vi "FuturePose.vi"(10 "IA State Input":T1) -> (2 "output cluster":T1={"our_robots"=[], "enemy_robots"=[], "balls"=[], "geometry"={"line_width"=0, "field_length"=0, "field_width"=0, "boundary_width"=0, "referee_width"=0, "goal_width"=0, "goal_depth"=0, "goal_wall_width"=0, "center_circle_radius"=0, "defense_radius"=0, "defense_stretch"=0, "free_kick_from_defense_dist"=0, "penalty_spot_from_field_line_dist"=0, "penalty_line_from_spot_dist"=0}, "IA Judge"={"stage"="", "command"="", "our_goalie_id"=0.0, "enemy_goalie_id"=0.0, "command enum"=enum."Halt", "Time"=enum."Azul"}, "Received Timestamp"=timestamp(0 s since 1904-01-01), "Events"={"Touch"=FALSE, "Ball out"=FALSE, "id touch"=0.0, "Ball out of \nVision"=FALSE, "Ball inside \nGoalie area"=FALSE, "Robot not responding"=FALSE, "Robots responding status"=[1.0, 1.0, 1.0, 1.0, 1.0, 1.0], "Enemy Ball \nPossession"=FALSE, "Pass State"=FALSE, "id end of pass"=0.0, "Kick"=FALSE, "Id ini Possession"=0.0, "Ball Possesion"=FALSE, "Id Possesion"=0.0, "Direct Kick"=FALSE, "2nd Strk Ativo"=FALSE}})   [LabVIEW 2020]
uses:
  SSL Detection Frame Simple Estimator Cameras VelCmd Folder/Core/AI Input.ctl
  Controls/AI Robot.ctl
  Controls/Functions Enum.ctl
  Controls/AttackerStates.ctl
  Controls/PathDests.ctl
  Controls/PathDest.ctl
  SSL Detection Frame Simple Estimator Cameras VelCmd Folder/Core/AI Ball.ctl
  SSL Detection Frame Simple Estimator Cameras VelCmd Folder/Core/Field Size.ctl
  SSL Detection Frame Simple Estimator Cameras VelCmd Folder/Core/AI Judge.ctl
  Communication_class/Paths/MessageAI_State Folder/Intel/Command Enum.ctl
  SSL Detection Frame Simple Estimator Cameras VelCmd Folder/Util/Events/Events.ctl
  <vilib>/Analysis/coordinate.llb/2D Cartesian Coordinate Rotation (Scalar).vi
  <vilib>/Analysis/NI_AALPro.lvlib
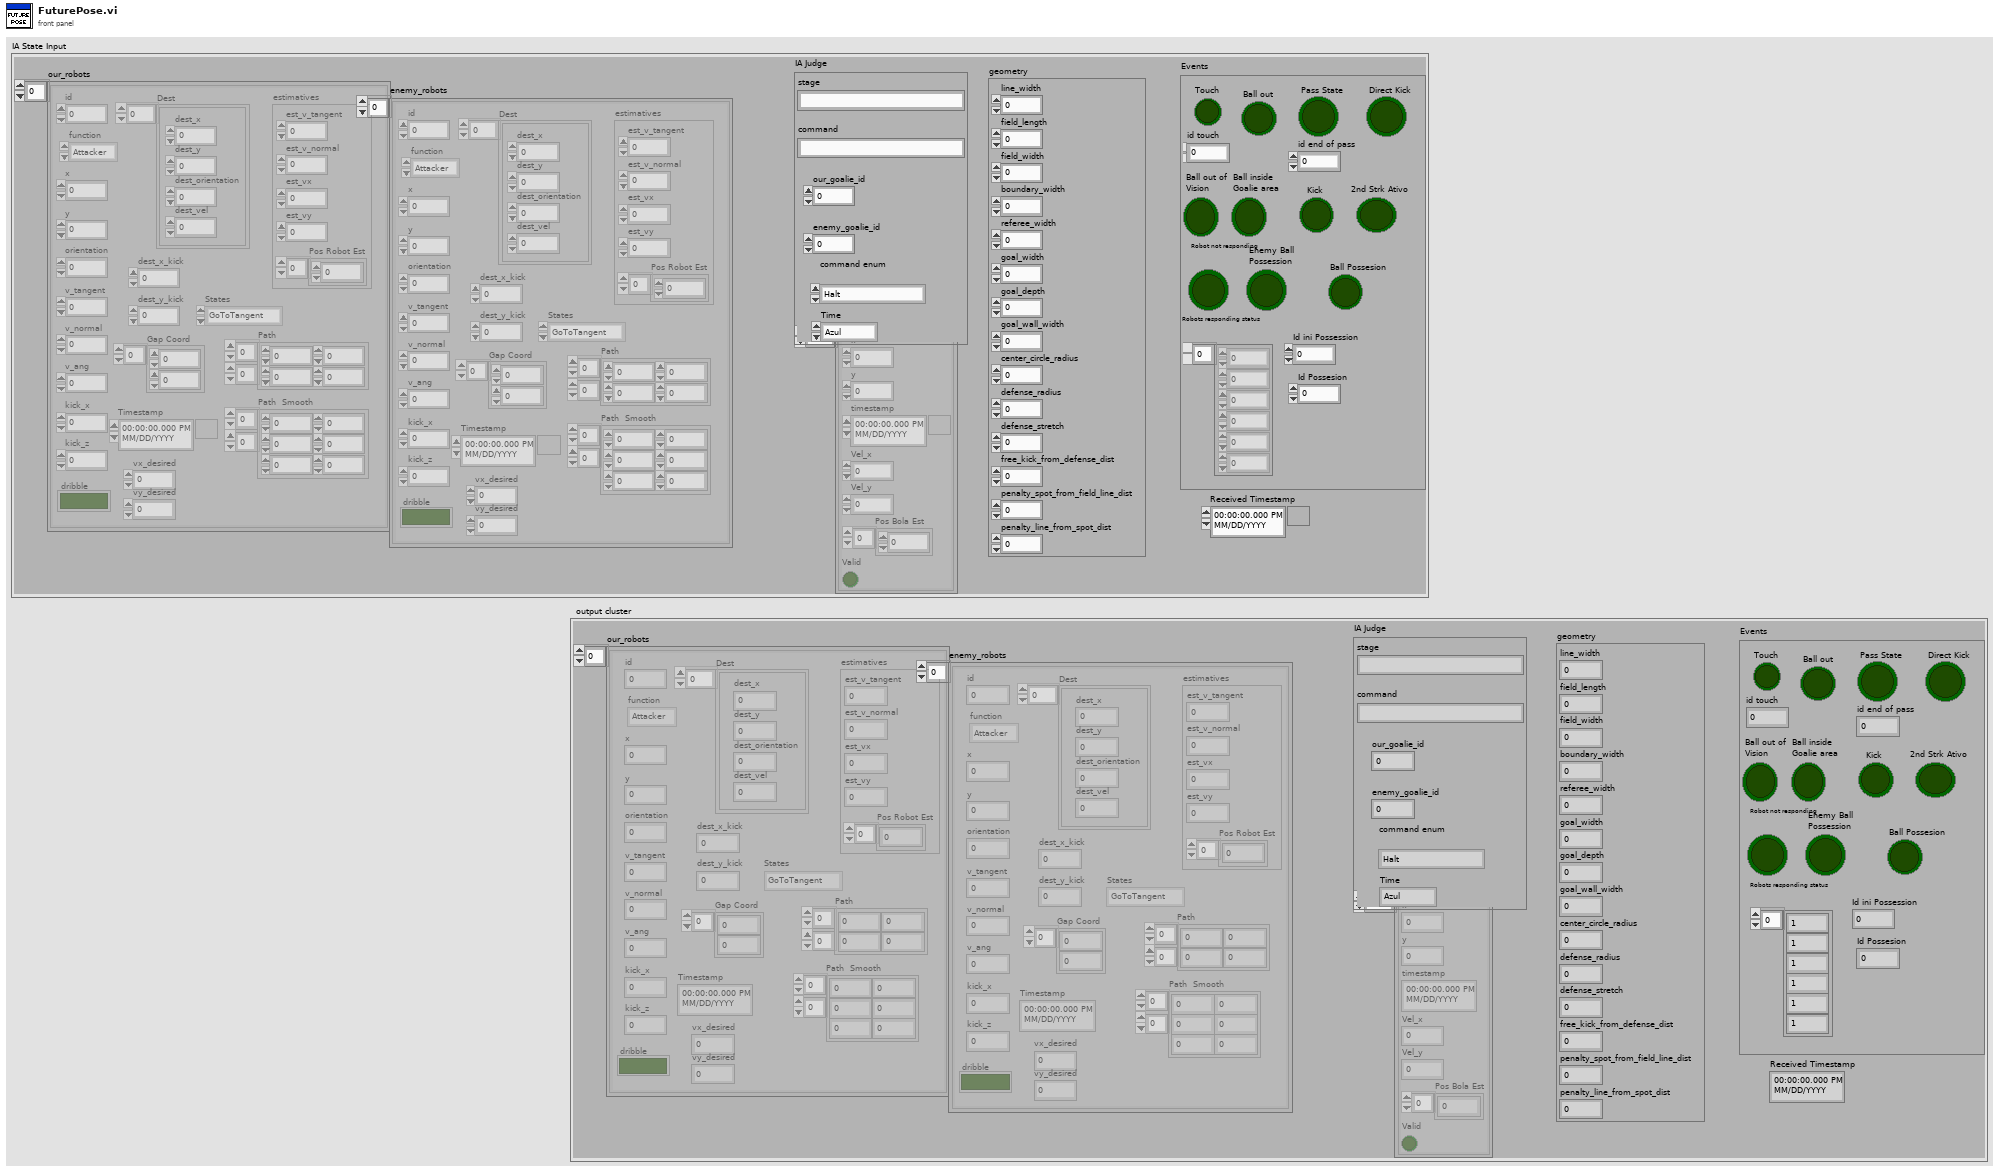
[diagram p1: front panel]
types:
  T1 = typedef "AI Input.ctl" = cluster{"our_robots":T2[], "enemy_robots":T2[], "balls":T7[], "geometry":T8, "IA Judge":T9, "Received Timestamp":timestamp, "Events":T11}
  T2 = typedef "AI Robot.ctl" = cluster{"id":u32, "function":T3, "x":dbl, "y":dbl, "orientation":dbl, "v_tangent":dbl, "v_normal":dbl, "v_ang":dbl, "kick_x":dbl, "kick_z":dbl, "dribble":bool, "Timestamp":timestamp, "estimatives":cluster{"est_v_tangent":dbl, "est_v_normal":dbl, "est_vx":dbl, "est_vy":dbl, "Pos Robot Est":dbl[]}, "dest_x_kick":dbl, "dest_y_kick":dbl, "Gap Coord":dbl[], "States":T4, "Path ":dbl[][], "Path  Smooth":dbl[][], "Dest":T5, "vx_desired":dbl, "vy_desired":dbl}
  T3 = typedef "Functions Enum.ctl" = enum16{"2nd Striker", "Attacker", "Goalie", "Defender", "Striker", "Goto 0", "Dummy", "Kicker", "ZigZag 0", "ZigZag 1", "ZigZag 2", "ZigZag 3", "ZigZag 4", "ZigZag 5", "ZigZag 6", "ZigZag 7", "ZigZag 8", ""}
  T4 = typedef "AttackerStates.ctl" = enum16{"Pass", "GoToTangent", "BallGetting", "GoToKick", ""}
  T5 = typedef "PathDests.ctl" = T6[]
  T6 = typedef "PathDest.ctl" = cluster{"dest_x":dbl, "dest_y":dbl, "dest_orientation":dbl, "dest_vel":dbl}
  T7 = typedef "AI Ball.ctl" = cluster{"x":dbl, "y":dbl, "timestamp":timestamp, "Vel_x":dbl, "Vel_y":dbl, "Pos Bola Est":dbl[], "Valid":bool}
  T8 = typedef "Field Size.ctl" = cluster{"line_width":u32, "field_length":u32, "field_width":u32, "boundary_width":u32, "referee_width":u32, "goal_width":u32, "goal_depth":u32, "goal_wall_width":u32, "center_circle_radius":u32, "defense_radius":u32, "defense_stretch":u32, "free_kick_from_defense_dist":u32, "penalty_spot_from_field_line_dist":u32, "penalty_line_from_spot_dist":u32}
  T9 = typedef "AI Judge.ctl" = cluster{"stage":string, "command":string, "our_goalie_id":dbl, "enemy_goalie_id":dbl, "command enum":T10, "Time":enum16{"Azul", "Amarelo"}}
  T10 = typedef "Command Enum.ctl" = enum16{"Halt", "Stop", "Force Start", "PKA Normal Start", "Prepare Kickoff Ally", "PKE Normal Start", "Prepare Kickoff Enemy", "Prepare Penalty Ally", "PPA Normal Start", "Prepare Penalty Enemy", "PPE Normal Start", "Direct Free Enemy", "Direct Free Ally", "Indirect Free Enemy", "Indirect Free Ally", "Timeout Enemy", "Timeout Ally", "Goal Enemy", "Goal Ally", "Ball Placement Enemy", "Ball Placement Ally", "Normal Half Time", "Extra Time Break", "Extra Half Time", "None", "Post Game"}
  T11 = typedef "Events.ctl" = cluster{"Touch":bool, "Ball out":bool, "id touch":dbl, "Ball out of \nVision":bool, "Ball inside \nGoalie area":bool, "Robot not responding":bool, "Robots responding status":dbl[], "Enemy Ball \nPossession":bool, "Pass State":bool, "id end of pass":dbl, "Kick":bool, "Id ini Possession":dbl, "Ball Possesion":bool, "Id Possesion":dbl, "Direct Kick":bool, "2nd Strk Ativo":bool}
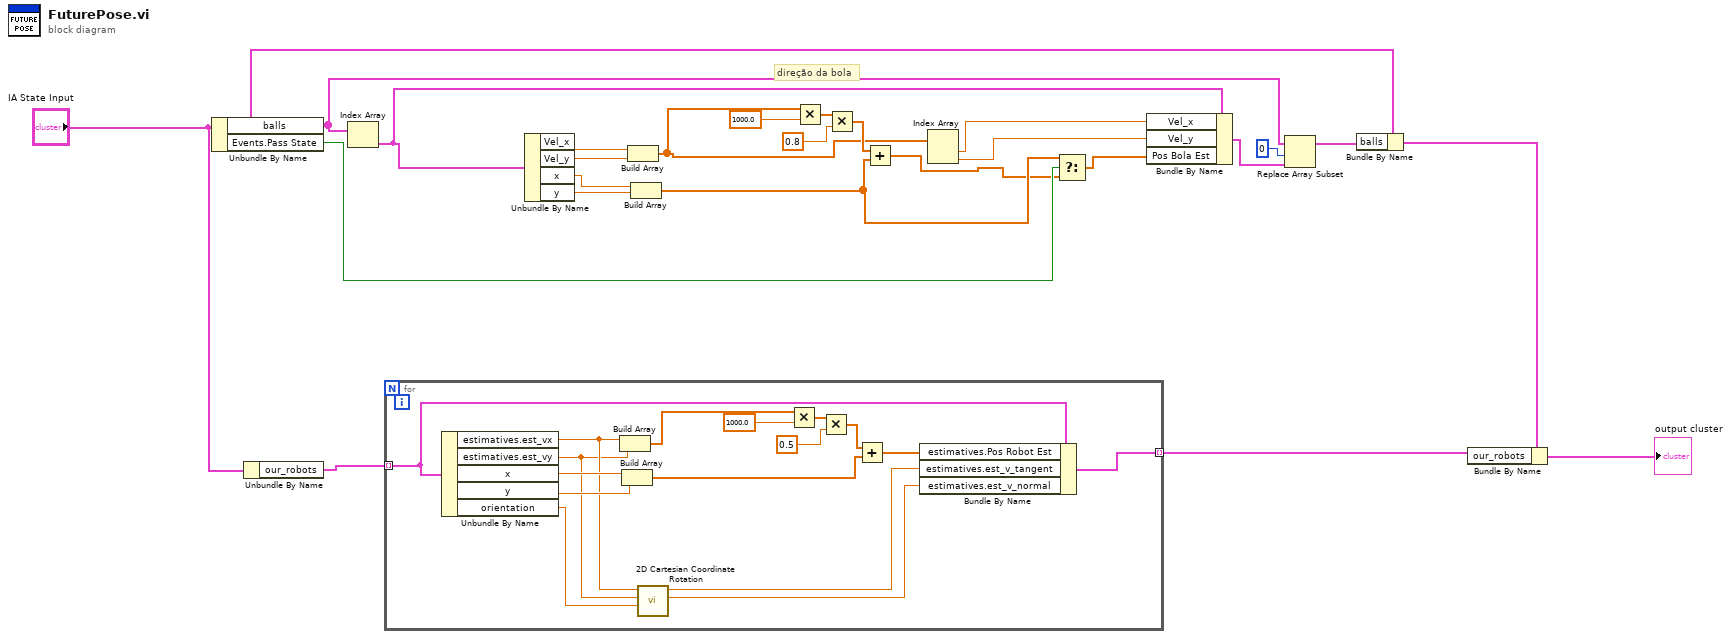
[diagram p0: block diagram]
diagram:
  # "direção da bola"
  n1 = Unbundle By Name("IA State Input") -> ("balls"=w21:T7[], "Events.Pass State"=w7:bool)
  n2 = Unbundle By Name("IA State Input") -> ("our_robots"=w6:T2[])
  n3 = Index Array(array=w21) -> (element=w23:T7)  [unwired: 1 in]
  n4 = for {
    tunnel: w6 -> [w33] mode=indexing
    tunnel: [w31] -> w5 mode=indexing
    n5 = Unbundle By Name(w33) -> ("estimatives.est_vx"=w30:dbl, "estimatives.est_vy"=w29:dbl, "x"=w35:dbl, "y"=w34:dbl, "orientation"=w28:dbl)
    n6 = Build Array(w30, w29) -> (w37:dbl[])
    n7 = Build Array(w35, w34) -> (w36:dbl[])
    n8 = call-poly <vilib>:"2D Cartesian Coordinate Rotation.vi"("theta"=w28, "y"=w29, "x"=w30) -> ("y out"=w26:dbl, "x out"=w27:dbl)  [unwired: 6 in, 1 out]
    n9 = Multiply(x=w37, y=1000.0) -> (x*y=w39:dbl[])
    n10 = Multiply(x=w39, y=0.5) -> (x*y=w40:dbl[])
    n11 = Add(x=w40, y=w36) -> (x+y=w32:dbl[])
    n12 = Bundle By Name(cluster=w33, "estimatives.Pos Robot Est"=w32, "estimatives.est_v_tangent"=w27, "estimatives.est_v_normal"=w26) -> (w31:T2)
  }
  n13 = Unbundle By Name(w23) -> ("Vel_x"=w25:dbl, "Vel_y"=w24:dbl, "x"=w18:dbl, "y"=w17:dbl)
  n14 = Build Array(w25, w24) -> (w4:dbl[])
  n15 = Build Array(w18, w17) -> (w9:dbl[])
  n16 = Multiply(x=w4, y=1000.0) -> (x*y=w15:dbl[])
  n17 = Multiply(x=w15, y=0.8) -> (x*y=w14:dbl[])
  n18 = Add(x=w14, y=w9) -> (x+y=w1:dbl[])
  n19 = Index Array(array=w4) -> (element #1=w3:dbl, element #2=w2:dbl)  [unwired: 2 in]
  n20 = Select(t=w9, s=w7, f=w1) -> (s? t:f=w8:dbl[])
  n21 = Bundle By Name(cluster=w23, "Vel_x"=w3, "Vel_y"=w2, "Pos Bola Est"=w8) -> (w20:T7)
  n22 = Replace Array Subset(array=w21, new element=w20, index=0) -> (w22:T7[])
  n23 = Bundle By Name(cluster="IA State Input", "balls"=w22) -> (w11:T1)
  n24 = Bundle By Name(cluster=w11, "our_robots"=w5) -> (→"output cluster":T1)
